vi "ConfigOutputMode.vi"(8 "error in (no error)":errorcluster, 11 "ClassIn":refnum<class "Keysight335XX.lvclass">) -> (0 "error out":errorcluster, 3 "ClassOut":refnum<class "Keysight335XX.lvclass">)   [LabVIEW 2014, in "FGenPlugins.lvlib" / "Keysight335XX.lvclass"]
uses:
  Keysight335XX.lvclass
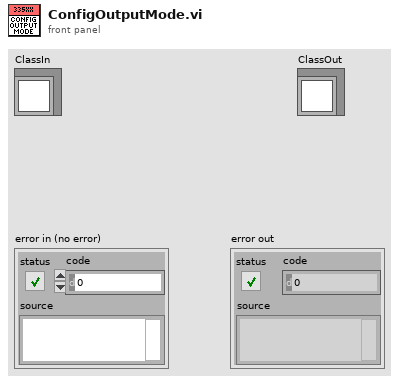
[diagram p1: front panel]
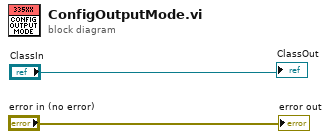
[diagram p0: block diagram]
diagram:
  "error out" <- "error in (no error)"
  "ClassOut" <- "ClassIn"
